vi "DegToRad.vi"(1 "deg":dbl) -> (0 "rad":dbl)   [LabVIEW 2018]
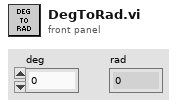
[diagram p1: front panel]
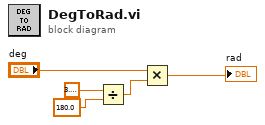
[diagram p0: block diagram]
diagram:
  n1 = Divide(x=3.141592653589793, y=180.0 ("x")) -> (x/y=w5:dbl)
  n2 = Multiply(x="deg", y=w5) -> (x*y=→"rad":dbl)
